vi "NewtonsPSM_Meas_Integra.vi"(0 "VISA session":refnum<visa-resource-name>, 9 "Stop":bool, 11 "error in (no error)":errorcluster) -> (4 "dup VISA session":refnum<visa-resource-name>, 6 "Read Strings":string, 8 "Measure":dbl[](array[numeric]) format="%^.4e", 15 "error out":errorcluster)   [LabVIEW 2025, in "NewtonsPSM1735.lvlib"]
doc: "This VI Start And Sop Integration and readback the integrator data from the PPA2530"
uses:
  NewtonsPSM1735.lvlib
panel:
  # "Wh"
  # "Wh,Fund"
  # "VAh"
  # "VAh,Fund"
  # "PF"
  # "PF,Fund"
  # "Ah"
  # "Ah, fund"
  # "Time"
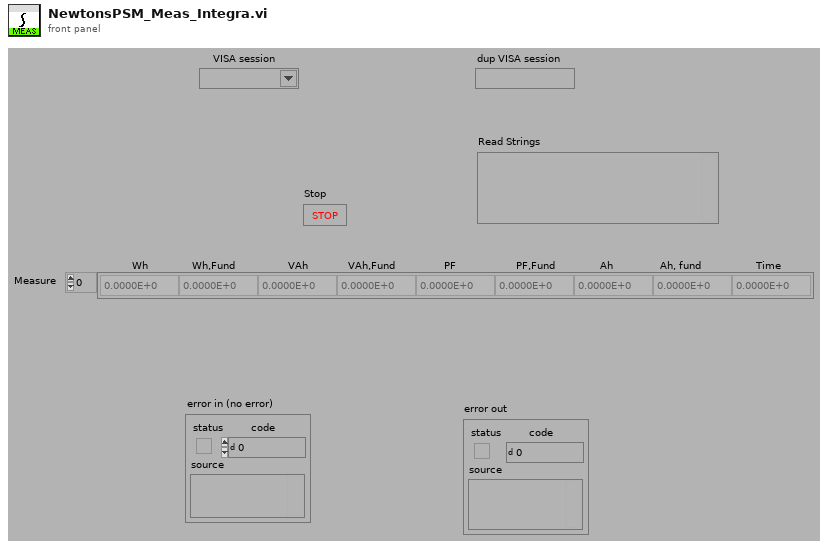
[diagram p1: front panel]
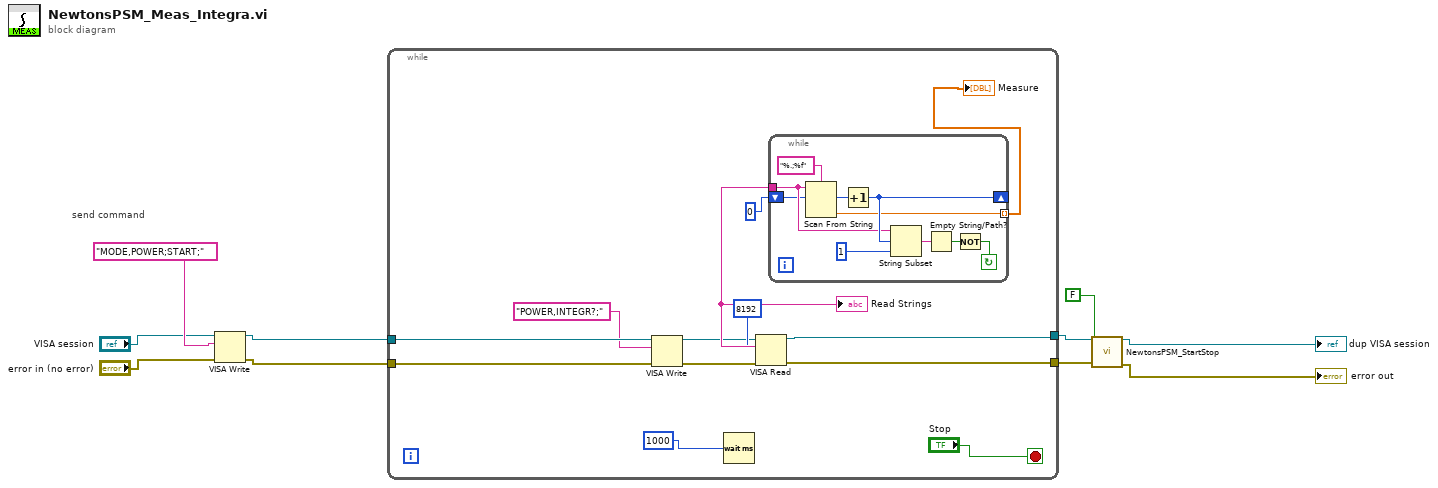
[diagram p0: block diagram]
diagram:
  # "send command"
  n1 = VISA Write(VISA resource name="VISA session", write buffer="MODE,POWER;START;", error in (no error)="error in (no error)") -> (VISA resource name out=w10:refnum<visa-resource-name>, error out=w9:errorcluster)  [unwired: 1 out]
  n2 = while {
    tunnel: w10 -> [w18]
    tunnel: w9 -> [w17]
    tunnel: [w16] -> w4
    tunnel: [w15] -> w5
    stop <- "Stop" stop-if-true
    n3 = VISA Write(VISA resource name=w18, write buffer="POWER,INTEGR?;", error in (no error)=w17) -> (VISA resource name out=w21:refnum<visa-resource-name>, error out=w20:errorcluster)  [unwired: 1 out]
    n4 = Wait (ms)(milliseconds to wait=1000) -> ()  [unwired: 1 out]
    n5 = VISA Read(VISA resource name=w21, byte count=u32 8192 ("ÊÞ²Ä¶³ÝÄi0j"), error in (no error)=w20) -> (VISA resource name out=w16:refnum<visa-resource-name>, read buffer=w23:string, error out=w15:errorcluster)  [unwired: 1 out]
    "Read Strings" <- w23
    n6 = while {
      tunnel: [w25] -> w12 mode=indexing
      shift-left: 0 -> [w24]
      shift-right: [w29] -> _
      tunnel: w23 -> [w27]
      stop <- w30 continue-if-true
      n7 = Scan From String(format string="%.;%f", input string=w27, initial scan location=w24) -> (offset past scan=w26:u32, output 1=w25:dbl)  [unwired: 1 in, 3 out]
      n8 = Increment(x=w26) -> (x+1=w29:u32)
      n9 = String Subset(string=w27, offset (0)=w29, length (rest)=1) -> (substring=w32:string)
      n10 = Empty String/Path?(string/path=w32) -> (empty?=w31:bool)
      n11 = Not(x=w31) -> (.not. x?=w30:bool)
    }
    "Measure" <- w12
  }
  n12 = call "NewtonsPSM_StartStop.vi"("VISA session"=w4, "Hold (F: ON)"=FALSE, "error in (no error)"=w5) -> ("dup VISA session"=→"dup VISA session":refnum<visa-resource-name>, "error out"=→"error out":errorcluster)  [unwired: 11 out]
